vi "Actor Core.vi"(8 "error in":errorcluster, 11 "Businness Logic in":refnum<class "Businness Logic.lvclass">) -> (0 "error out":errorcluster, 3 "Actor out":refnum<class "Actor.lvclass">)   [LabVIEW 2020, in "Businness Logic.lvlib" / "Businness Logic.lvclass"]
doc: "(<B>Filename</B>: Actor Framework.lvlib:Actor.lvclass:Actor Core.vi)\n\nReceives messages to the actor, reacts to them, and initiates any error handling that may shut the actor down.\n\nDescendant classes may override this VI to append parallel tasks for the actor to complete while it handles messages. Overrides use the Call Parent Class Method node."
uses:
  Businness Logic.lvclass
  C:/Program Files (x86)/National Instruments/LabVIEW 2020/vi.lib/ActorFramework/Actor/Actor.lvclass
  <vilib>/ActorFramework/Actor/Actor.lvclass
  Acquisition/Acquisition/Acquisition.lvclass
  Logging/Logging/Logging.lvclass
  User Interface/User Interface.lvclass
  Businness Logic.lvclass/Businness Logic.ctl
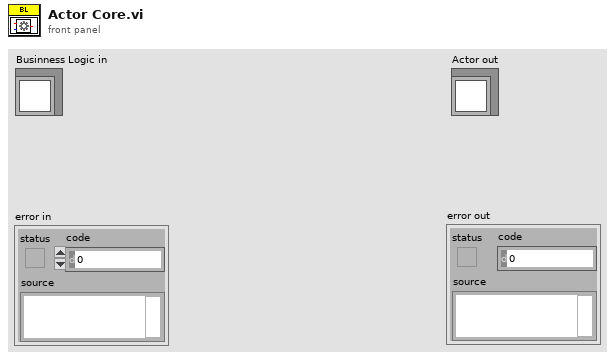
[diagram p1: front panel]
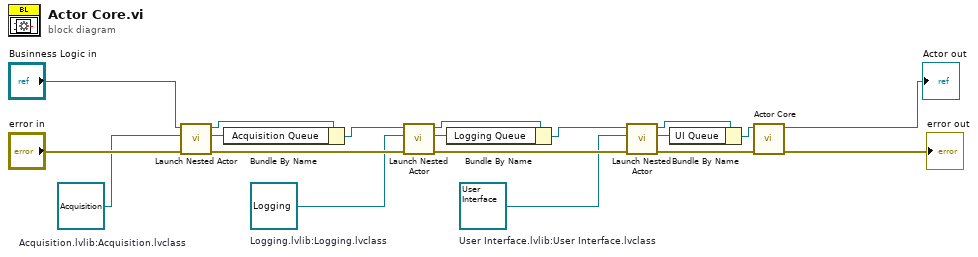
[diagram p0: block diagram]
diagram:
  w3 = refnum<class "User Interface.lvclass"> refnum  # User Interface.lvlib:User Interface.lvclass
  w4 = refnum<class "Logging.lvclass"> refnum  # Logging.lvlib:Logging.lvclass
  w5 = refnum<class "Acquisition.lvclass"> refnum  # Acquisition.lvlib:Acquisition.lvclass
  n1 = call <vilib>:"Launch Nested Actor.vi"("error in (no error)"="error in", "Nested Actor"=w5, "Caller Actor in"="Businness Logic in") -> ("error out"=w13:errorcluster, "Nested Actor's Enqueuer"=w9:refnum<class "Message Enqueuer.lvclass">, "Caller Actor out"=w11:refnum<class "Businness Logic.lvclass">)  [unwired: 6 in]
  n2 = Bundle By Name(cluster=w11, "Acquisition Queue"=w9) -> (w10:refnum<class "Businness Logic.lvclass">)
  n3 = call <vilib>:"Launch Nested Actor.vi"("error in (no error)"=w13, "Nested Actor"=w4, "Caller Actor in"=w10) -> ("error out"=w16:errorcluster, "Nested Actor's Enqueuer"=w7:refnum<class "Message Enqueuer.lvclass">, "Caller Actor out"=w15:refnum<class "Businness Logic.lvclass">)  [unwired: 6 in]
  n4 = Bundle By Name(cluster=w15, "Logging Queue"=w7) -> (w8:refnum<class "Businness Logic.lvclass">)
  n5 = call <vilib>:"Launch Nested Actor.vi"("error in (no error)"=w16, "Nested Actor"=w3, "Caller Actor in"=w8) -> ("error out"=w1:errorcluster, "Nested Actor's Enqueuer"=w2:refnum<class "Message Enqueuer.lvclass">, "Caller Actor out"=w14:refnum<class "Businness Logic.lvclass">)  [unwired: 6 in]
  n6 = Bundle By Name(cluster=w14, "UI Queue"=w2) -> (w6:refnum<class "Businness Logic.lvclass">)
  n7 = call-parent "Actor Core.vi"("error in"=w1, "Actor in"=w6) -> ("error out"=→"error out":errorcluster, "Actor out"=→"Actor out":refnum<class "Actor.lvclass">)  [unwired: 8 in]
